vi "Wrapper.vi"(8 "error in (no error)":errorcluster, 10 "Actor in":refnum<class "Actor.lvclass">, 11 "O3 Valve in":refnum<class "O3 Valve MSG.lvclass">) -> (0 "error out":errorcluster, 3 "Controller out":refnum<class "Controller.lvclass">)   [LabVIEW 2015, in "Controller.lvlib" / "O3 Valve MSG.lvclass"]
uses:
  O3 Valve MSG.lvclass
  Controller.lvclass
  <vilib>/ActorFramework/Actor/Actor.lvclass
  Update Switch State MSG/Update Switch MSG.lvclass/Update Switch MSG.ctl
  SuperActor/SuperActor.lvclass/SuperActor.ctl
  <vilib>/DAQmx/write.llb/DAQmx Write (Digital Bool 1Line 1Point).vi
  Update Switch State MSG/Read SwitchState.vi
  SuperActor/Read Log Session.vi
  SuperActor/Read CVT Session.vi
  <vilib>/DAQmx/miscellaneous.llb/DAQmx Fill In Error Info.vi
  <vilib>/MSR Consulting, LLC/ESF/Session - Root.lvclass
  reusable/Session APIs/Session Log/System Log.lvclass
  reusable/Session APIs/CVT/CVT.lvclass
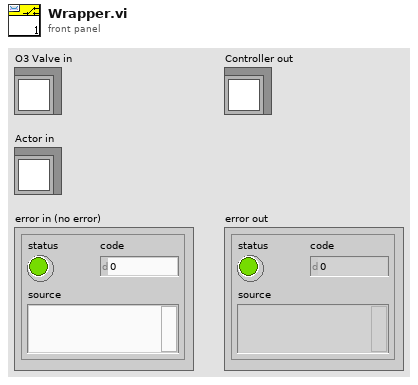
[diagram p1: front panel]
types:
  T1 = typedef "Session - Root.lvclass/Session Handle.ctl" = refnum<data-value>
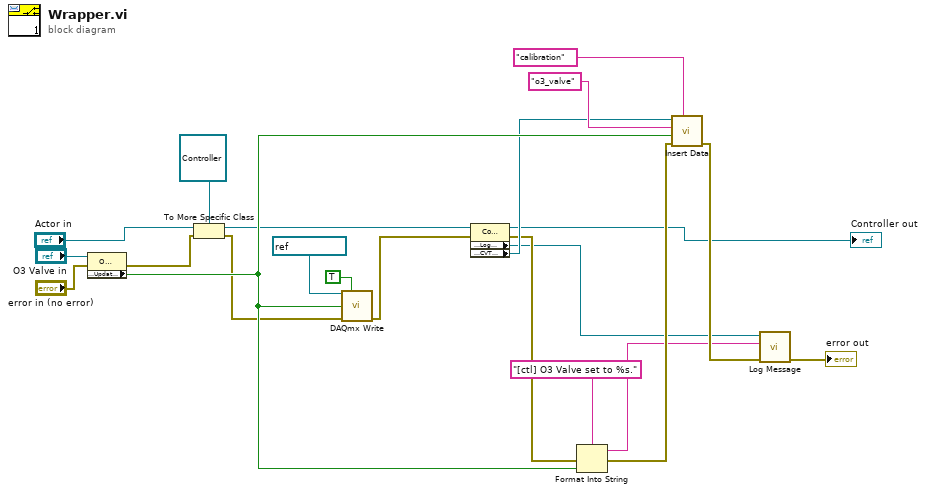
[diagram p0: block diagram]
diagram:
  n1 = property class="O3 Valve"(reference="O3 Valve in", error in="error in (no error)") -> (error out=w16:errorcluster, "Accessors:UpdateSw"=w20:bool)  [unwired: 1 out]
  n2 = To More Specific Class(target class=refnum<class "Controller.lvclass"> refnum ("Controller.lvlib:Controller"), reference="Actor in", error in=w16) -> (specific class reference=w6:refnum<class "Controller.lvclass">, error out=w5:errorcluster)
  n3 = call-poly <vilib>:"DAQmx Write.vi"("task/channels in"=refnum<k21> "O3 Valve", "auto start"=TRUE, "data"=w20, "error in"=w5) -> ("error out"=w7:errorcluster)  [unwired: 9 in, 2 out]
  n4 = property class="Controller"(reference=w6, error in=w7) -> (reference out=→"Controller out":refnum<class "Controller.lvclass">, error out=w10:errorcluster, "Accessors:Log Session"=w8:T1, "Accessors:CVT Session"=w17:T1)
  n5 = Format Into String(format string="[ctl] O3 Valve set to %s.", error in=w10, w20) -> (resulting string=w13:string, error out=w21:errorcluster)  [unwired: 1 in]
  n6 = call "Insert Data.vi"("Group"="calibration", "error in"=w21, "Data"=w20, "tag"="o3_valve", "CVT Session In"=w17) -> ("error out"=w22:errorcluster)  [unwired: 5 in, 1 out]
  n7 = call "Log Message.vi"("error in"=w22, "MSG In"=w13, "session in"=w8) -> ("error out"=→"error out":errorcluster)  [unwired: 7 in, 1 out]
